vi "Enum to Board Design.vi"(1 "which board":T1) -> (0 "board.lvclass":refnum<class "Board Design.lvclass">)   [LabVIEW 2023, in "Board Design.lvclass"]
doc: "Produce an object of the appropriate type, based on the kind of board."
uses:
  Board Design.lvclass
  Common/Board Type Enum.ctl
  DAQBasic/Basic DAQ Design.lvclass
  c:/dev/_r/4/eng/lv-core/lvpostprocessingd/lv_mc_x86_64/dist_i386/examples/Object-Oriented Programming/Board Testing/Object Design/Board/Board Design.lvclass
  DAQElite/Elite DAQ Design.lvclass
  GPIBBoard/GPIB Board Design.lvclass
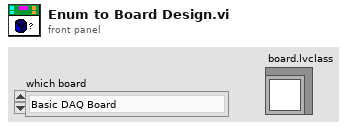
[diagram p1: front panel]
types:
  T1 = typedef "Board Type Enum.ctl" = enum16{"Basic DAQ Board", "Elite DAQ Board", "GPIB Board"}
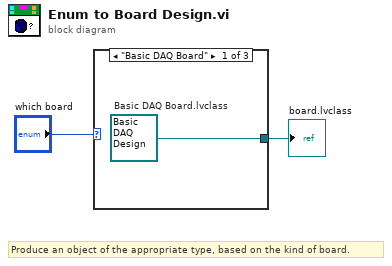
[diagram p0: block diagram]
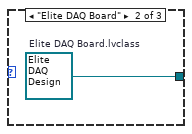
[diagram p2: hidden frame]
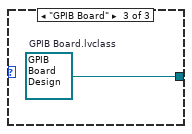
[diagram p3: hidden frame]
diagram:
  # "Produce an object of the appropriate type, based on the kind of board."
  n1 = case shown="\"Basic DAQ Board\"" "which board" {
    tunnel: [w3 w4 w5] -> w1
    frame "Basic DAQ Board" {
      w3 = refnum<class "Basic DAQ Design.lvclass"> refnum  # Basic DAQ Board.lvclass
    }
    frame "Elite DAQ Board" {
      w4 = refnum<class "Elite DAQ Design.lvclass"> refnum  # Elite DAQ Board.lvclass
    }
    frame "GPIB Board" {
      w5 = refnum<class "GPIB Board Design.lvclass"> refnum  # GPIB Board.lvclass
    }
  }
  "board.lvclass" <- w1
